vi "objectOnBlock.vi"() -> ()   [LabVIEW 2015]
panel:
  out "error out":errorcluster
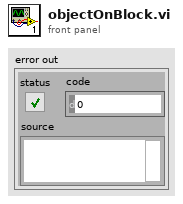
[diagram p1: front panel]
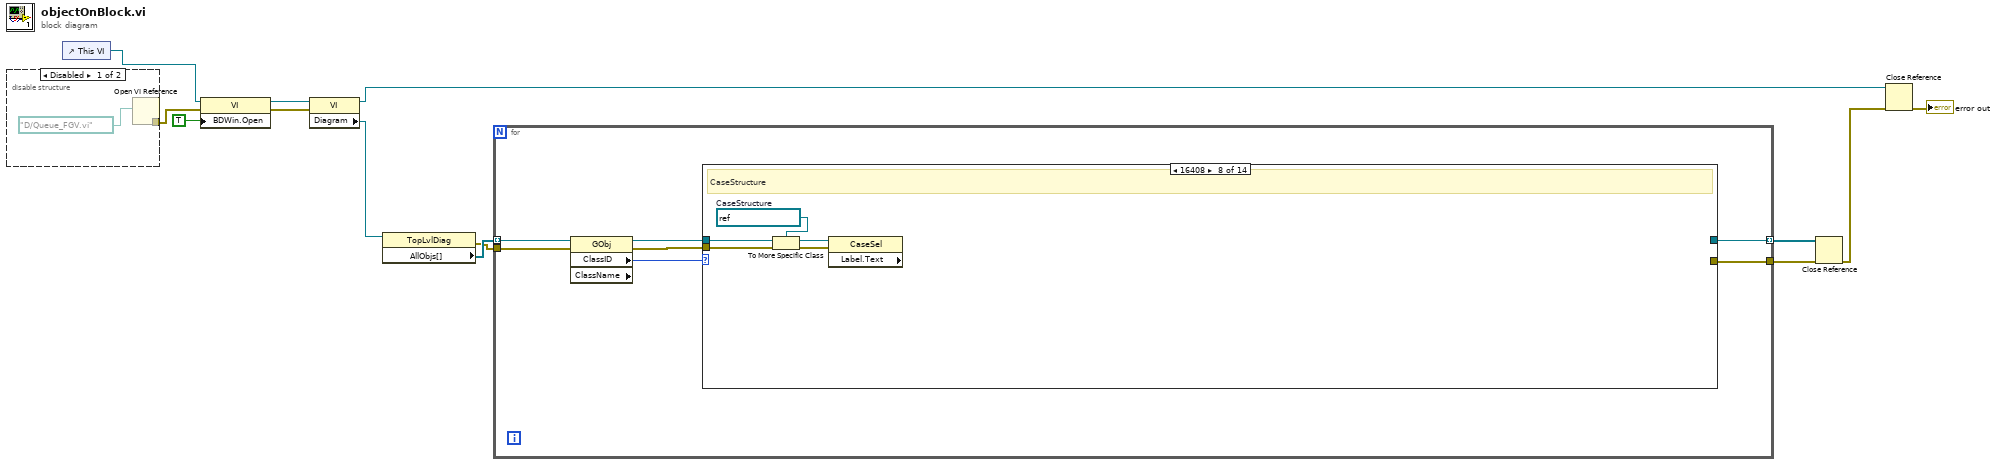
[diagram p0: block diagram]
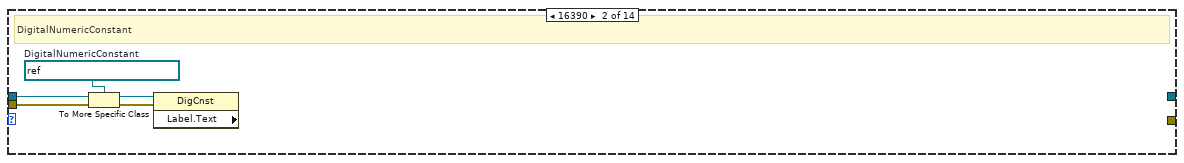
[diagram p4: hidden frame]
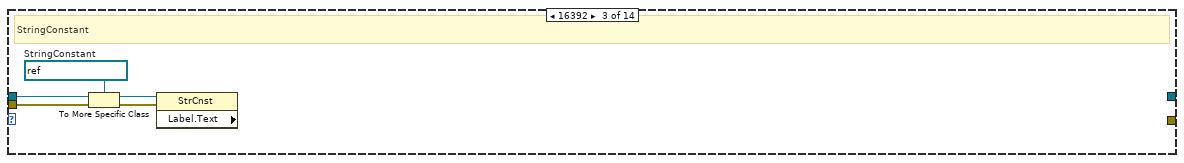
[diagram p5: hidden frame]
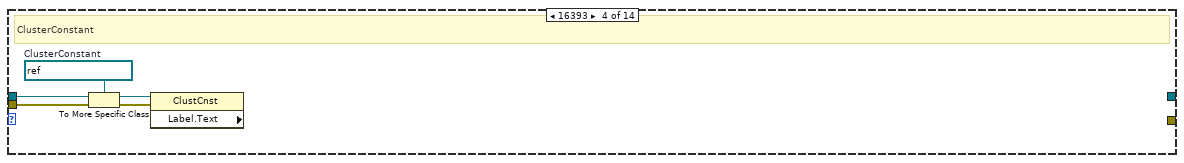
[diagram p6: hidden frame]
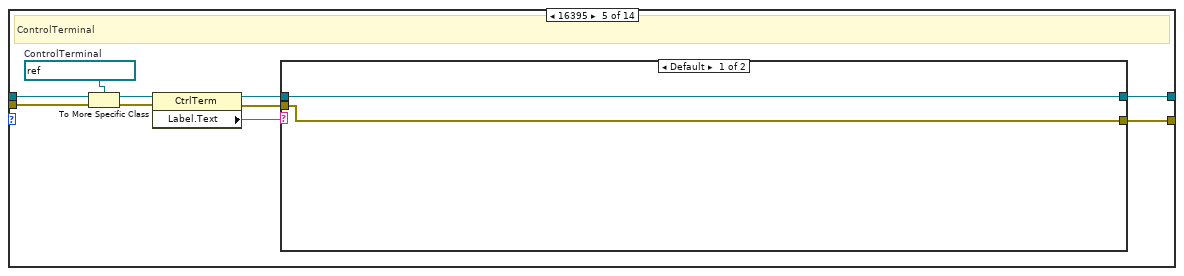
[diagram p7: hidden frame]
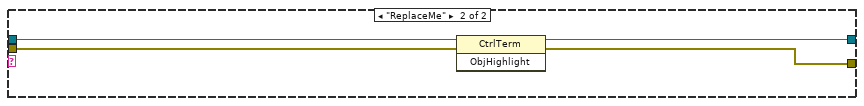
[diagram p8: hidden frame]
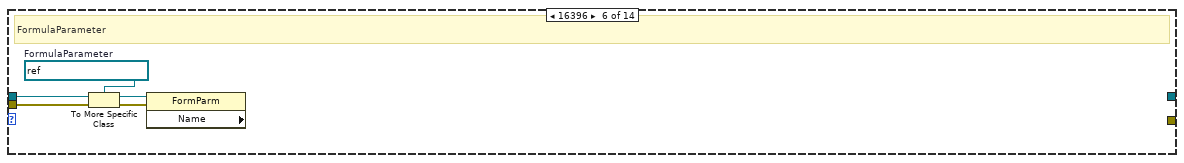
[diagram p9: hidden frame]
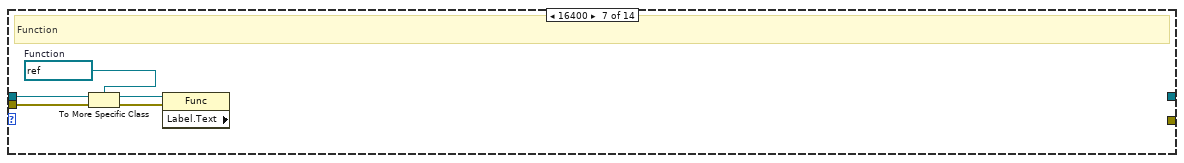
[diagram p10: hidden frame]
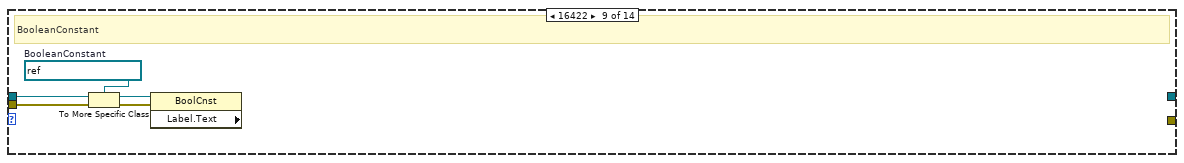
[diagram p11: hidden frame]
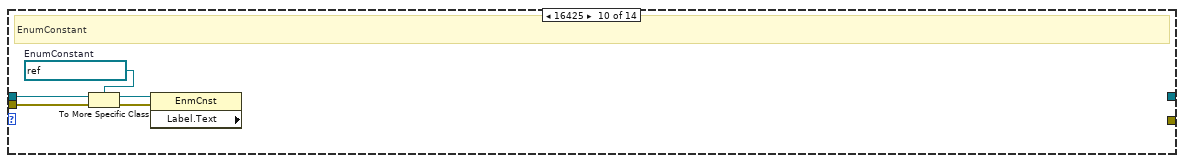
[diagram p12: hidden frame]
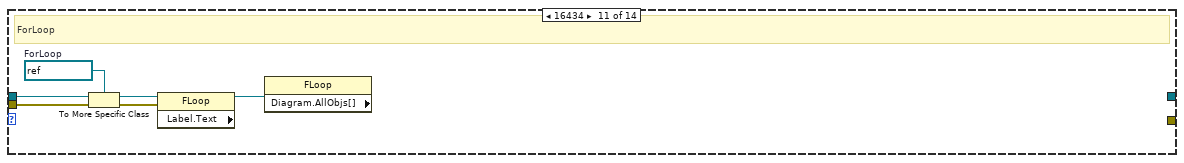
[diagram p13: hidden frame]
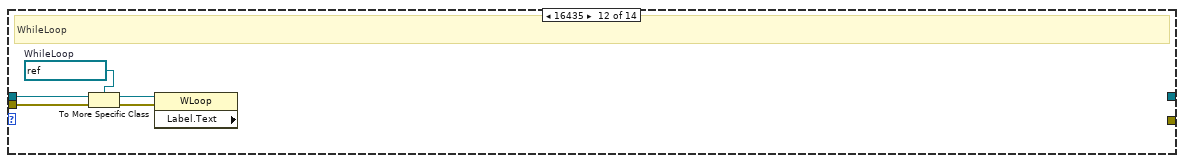
[diagram p14: hidden frame]
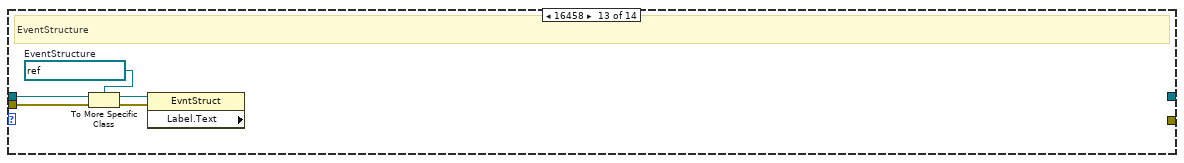
[diagram p15: hidden frame]
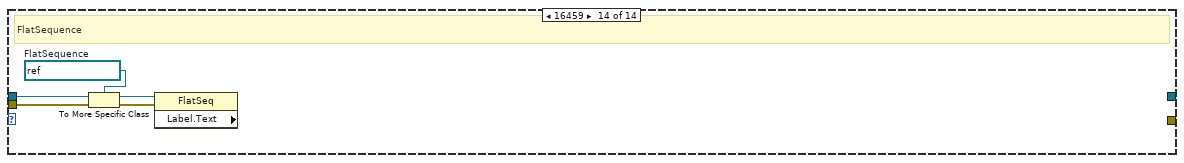
[diagram p16: hidden frame]
diagram:
  n1 = disable-structure shown="Disabled" {
    disable-tunnel: [w14 _] -> w13
    frame Disabled {
      n2 = Open VI Reference(vi path=path "D:/Queue_FGV.vi") -> (error out=w14:errorcluster)  [unwired: 5 in, 1 out]
    }
    frame Enabled {
    }
  }
  n3 = control-ref of="This VI"() -> (w2:refnum<vi>)
  n4 = property class="VI"(reference=w2, error in=w13, "BDWin.Open"=TRUE ("Block Diagram Window:Open")) -> (reference out=w11:refnum<vi>, error out=w1:errorcluster)
  n5 = property class="VI"(reference=w11, error in=w1) -> (reference out=w8:refnum<vi>, "Diagram"=w4:refnum<vi>)  [unwired: 1 out]
  n6 = property class="TopLvlDiag"(reference=w4) -> (error out=w3:errorcluster, "AllObjs[]"=w10:refnum<vi>[])  [unwired: 1 in, 1 out]
  n7 = for {
    tunnel: w10 -> [w22] mode=indexing
    tunnel: [w19] -> w9 mode=indexing
    tunnel: [w18] -> w6
    tunnel: w3 -> [w16]
    n8 = property class="GObj" props=["ClassID", "ClassName"](reference=w22, error in=w16) -> (reference out=w20:refnum<vi>, error out=w17:errorcluster, "ClassID"=w21:u32)  [unwired: 1 out]
    n9 = case shown="16408" w21 {
      tunnel: w20 -> [w24 w26 w32 w36 w49 w59 w64 w69 w72 w79 w85 w90 w95 w100]
      tunnel: [w24 _ _ _ w43 _ _ _ _ _ _ _ _ _] -> w19
      tunnel: [w23 _ _ _ w42 _ _ _ _ _ _ _ _ _] -> w18
      tunnel: w17 -> [w23 w25 w31 w35 w40 w58 w63 w68 w71 w78 w84 w89 w94 w99]
      frame 0, Default {
      }
      frame 16390 {
        w29 = refnum<vi> refnum  # DigitalNumericConstant
        # "DigitalNumericConstant"
        n10 = To More Specific Class(target class=w29, reference=w26, error in=w25) -> (specific class reference=w28:refnum<vi>, error out=w27:errorcluster)
        n11 = property class="DigCnst" props=["Label", "Text"](reference=w28, error in=w27) -> ()  [unwired: 3 out]
      }
      frame 16392 {
        w33 = refnum<vi> refnum  # StringConstant
        # "StringConstant"
        n12 = To More Specific Class(target class=w33, reference=w32, error in=w31) -> (specific class reference=w30:refnum<vi>, error out=w34:errorcluster)
        n13 = property class="StrCnst" props=["Label", "Text"](reference=w30, error in=w34) -> ()  [unwired: 3 out]
      }
      frame 16393 {
        w38 = refnum<vi> refnum  # ClusterConstant
        # "ClusterConstant"
        n14 = To More Specific Class(target class=w38, reference=w36, error in=w35) -> (specific class reference=w37:refnum<vi>, error out=w39:errorcluster)
        n15 = property class="ClustCnst" props=["Label", "Text"](reference=w37, error in=w39) -> ()  [unwired: 3 out]
      }
      frame 16395 {
        w48 = refnum<vi> refnum  # ControlTerminal
        # "ControlTerminal"
        n16 = To More Specific Class(target class=w48, reference=w49, error in=w40) -> (specific class reference=w47:refnum<vi>, error out=w46:errorcluster)
        n17 = property class="CtrlTerm"(reference=w47, error in=w46) -> (reference out=w44:refnum<vi>, error out=w41:errorcluster, "Label.Text"=w45:string)
        n18 = case shown="Default" w45 {
          tunnel: w44 -> [w51 w53]
          tunnel: [w51 w55] -> w43
          tunnel: [w50 w54] -> w42
          tunnel: w41 -> [w50 w52]
          frame Default {
          }
          frame "ReplaceMe" {
            n19 = invoke class="CtrlTerm" method="ObjHighlight"(reference=w53, error in=w52) -> (reference out=w55:refnum<vi>, error out=w54:errorcluster)  [unwired: 1 in, 1 out]
          }
        }
      }
      frame 16396 {
        w57 = refnum<vi> refnum  # FormulaParameter
        # "FormulaParameter"
        n20 = To More Specific Class(target class=w57, reference=w59, error in=w58) -> (specific class reference=w56:refnum<vi>, error out=w60:errorcluster)
        n21 = property class="FormParm" props=["Name"](reference=w56, error in=w60) -> ()  [unwired: 3 out]
      }
      frame 16400 {
        w62 = refnum<vi> refnum  # Function
        # "Function"
        n22 = To More Specific Class(target class=w62, reference=w64, error in=w63) -> (specific class reference=w61:refnum<vi>, error out=w65:errorcluster)
        n23 = property class="Func" props=["Label", "Text"](reference=w61, error in=w65) -> ()  [unwired: 3 out]
      }
      frame 16408 {
        w67 = refnum<vi> refnum  # CaseStructure
        # "CaseStructure"
        n24 = To More Specific Class(target class=w67, reference=w69, error in=w68) -> (specific class reference=w66:refnum<vi>, error out=w70:errorcluster)
        n25 = property class="CaseSel" props=["Label", "Text"](reference=w66, error in=w70) -> ()  [unwired: 3 out]
      }
      frame 16422 {
        w74 = refnum<vi> refnum  # BooleanConstant
        # "BooleanConstant"
        n26 = To More Specific Class(target class=w74, reference=w72, error in=w71) -> (specific class reference=w73:refnum<vi>, error out=w75:errorcluster)
        n27 = property class="BoolCnst" props=["Label", "Text"](reference=w73, error in=w75) -> ()  [unwired: 3 out]
      }
      frame 16425 {
        w77 = refnum<vi> refnum  # EnumConstant
        # "EnumConstant"
        n28 = To More Specific Class(target class=w77, reference=w79, error in=w78) -> (specific class reference=w76:refnum<vi>, error out=w80:errorcluster)
        n29 = property class="EnmCnst" props=["Label", "Text"](reference=w76, error in=w80) -> ()  [unwired: 3 out]
      }
      frame 16434 {
        w83 = refnum<vi> refnum  # ForLoop
        # "ForLoop"
        n30 = To More Specific Class(target class=w83, reference=w85, error in=w84) -> (specific class reference=w82:refnum<vi>, error out=w86:errorcluster)
        n31 = property class="FLoop" props=["Label", "Text"](reference=w82, error in=w86) -> (reference out=w81:refnum<vi>)  [unwired: 2 out]
        n32 = property class="FLoop" props=["Diagram", "AllObjs[]"](reference=w81) -> ()  [unwired: 1 in, 3 out]
      }
      frame 16435 {
        w88 = refnum<vi> refnum  # WhileLoop
        # "WhileLoop"
        n33 = To More Specific Class(target class=w88, reference=w90, error in=w89) -> (specific class reference=w87:refnum<vi>, error out=w91:errorcluster)
        n34 = property class="WLoop" props=["Label", "Text"](reference=w87, error in=w91) -> ()  [unwired: 3 out]
      }
      frame 16458 {
        w93 = refnum<vi> refnum  # EventStructure
        # "EventStructure"
        n35 = To More Specific Class(target class=w93, reference=w95, error in=w94) -> (specific class reference=w92:refnum<vi>, error out=w96:errorcluster)
        n36 = property class="EvntStruct" props=["Label", "Text"](reference=w92, error in=w96) -> ()  [unwired: 3 out]
      }
      frame 16459 {
        w98 = refnum<vi> refnum  # FlatSequence
        # "FlatSequence"
        n37 = To More Specific Class(target class=w98, reference=w100, error in=w99) -> (specific class reference=w97:refnum<vi>, error out=w101:errorcluster)
        n38 = property class="FlatSeq" props=["Label", "Text"](reference=w97, error in=w101) -> ()  [unwired: 3 out]
      }
    }
  }
  n39 = Close Reference(reference=w9, error in (no error)=w6) -> (error out=w7:errorcluster)
  n40 = Close Reference(reference=w8, error in (no error)=w7) -> (error out=→"error out":errorcluster)
